vi "FP Server Repository.vi"(0 "FP Management In":refnum<class "Front Panel Manager.lvclass">, 5 "Action(ReadRepository)":T1(ring), 11 "error in (no error)":errorcluster) -> (4 "FP Management Out":refnum<class "Front Panel Manager.lvclass">, 6 "ToProcessQueue":refnum<queue>, 8 "ProcessAlreadyStarted":bool, 12 "ProcessViRef":refnum<vi>, 13 "ProcessSyncQueue":refnum<queue>, 14 "FromProcessQueue":refnum<queue>, 15 "error out":errorcluster)   [LabVIEW 2017, in "Front Panel Publisher.lvlib" / "Front Panel Manager.lvclass"]
uses:
  Front Panel Manager.lvclass
  FP Server Message.ctl
  FP Server.ctl
  Front Panel Manager.lvclass/Front Panel Manager.ctl
panel:
  # "Use this indicator for sending messages to the Process VI"
  # "These indicators are used by the process VIs"
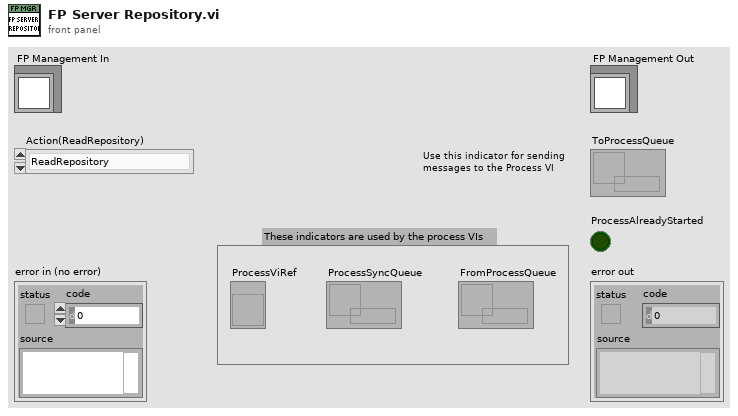
[diagram p1: front panel]
types:
  T1 = enum16{"ReadRepository", "CreateNew", "CreateOrLookUpExisting", "ReadRepositoryAndDestroy"}
  T2 = typedef "Front Panel Publisher.lvlib/Front Panel Manager.lvclass/FP Server.ctl" = cluster{"ToProcessQueue":refnum<queue>, "FromProcessQueue":refnum<queue>, "ProcessSyncQueue":refnum<queue>, "ProcessViRef":refnum<vi>}
  T3 = typedef "Front Panel Publisher.lvlib/Front Panel Manager.lvclass/FP Server Message.ctl" = cluster{"Message":string, "Page":string, "Data":string[][], "Connection ID":u64, "Values and Position":refnum<vi>[]}
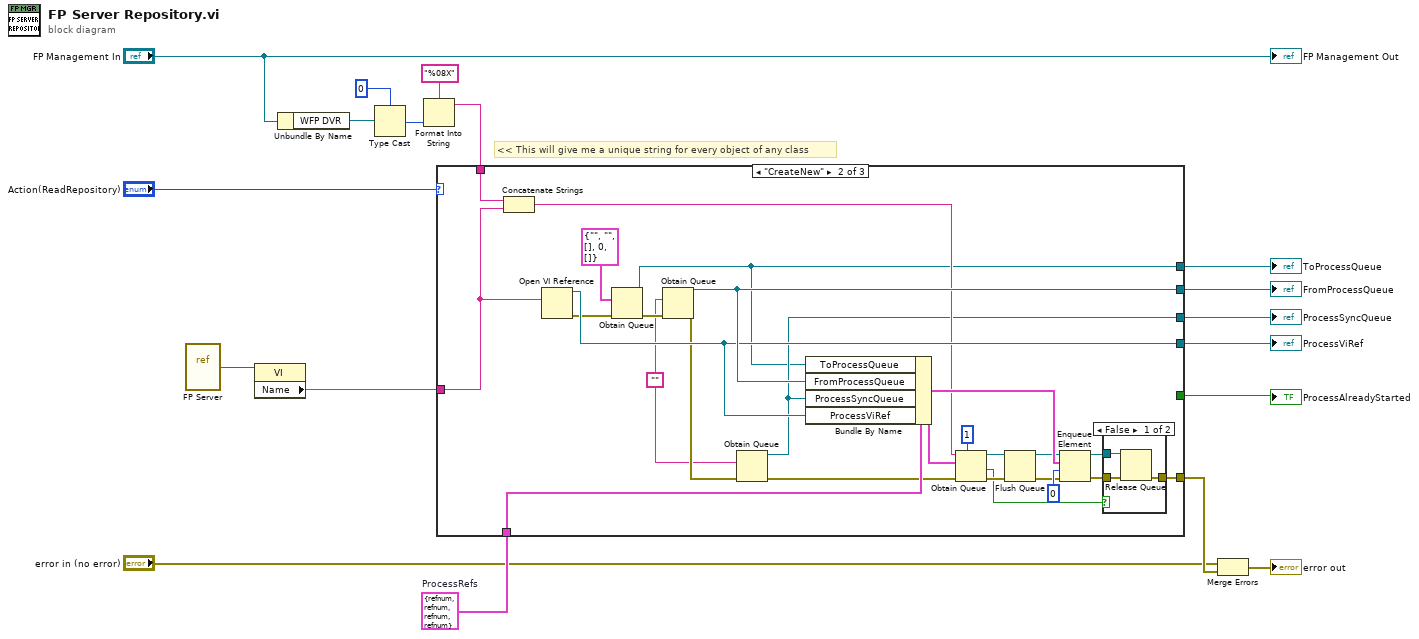
[diagram p0: block diagram]
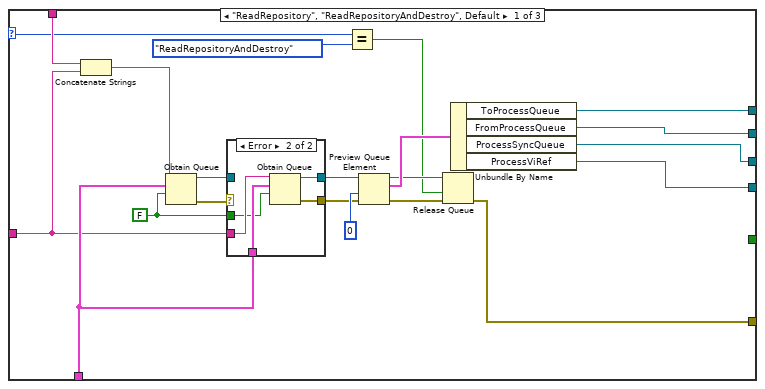
[diagram p2: hidden frame]
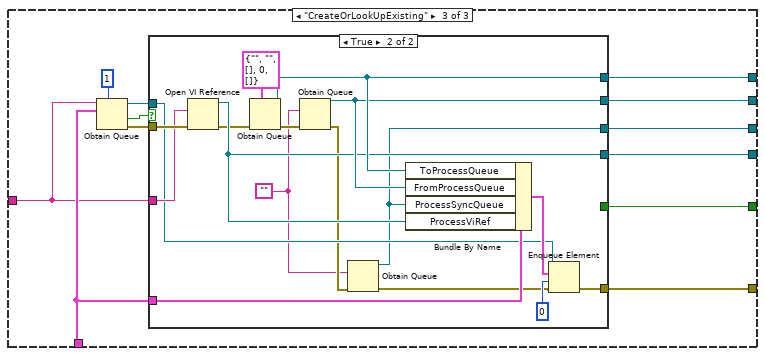
[diagram p5: hidden frame]
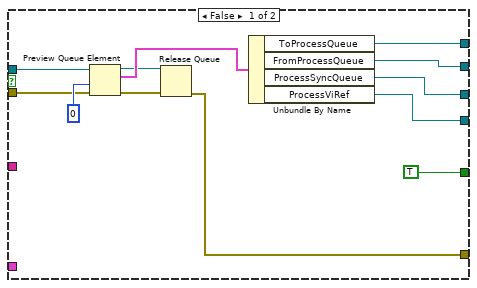
[diagram p6: hidden frame]
diagram:
  w13 = T2 {"ToProcessQueue"=refnum, "FromProcessQueue"=refnum, "ProcessSyncQueue"=refnum, "ProcessViRef"=refnum}  # ProcessRefs
  # "<< This will give me a unique string for every object of any class"
  n1 = vi-ref "FP Server.vi"() -> (w1:refnum<vi>)
  n2 = property class="VI"(reference=w1) -> ("Name"=w2:string)  [unwired: 1 in, 2 out]
  n3 = Unbundle By Name("FP Management In") -> ("WFP DVR"=w3:refnum<data-value>)
  n4 = Type Cast(type=u32 0, x=w3) -> (*(type *) &x=w8:u32)
  n5 = Format Into String(format string="%08X", w8) -> (resulting string=w5:string)  [unwired: 2 in, 1 out]
  n6 = case shown="\"CreateNew\"" "Action(ReadRepository)" {
    selector: "Action(ReadRepository)" -> [w20 _ _]
    tunnel: [w34 w57 w85] -> w17
    tunnel: [w36 w47 w87] -> w15
    tunnel: [w35 w71 w86] -> w16
    tunnel: [w37 w70 w84] -> w14
    tunnel: w13 -> [w29 w63 w80]
    tunnel: w5 -> [w27 w62 _]
    tunnel: [w22 w50 w83] -> w11
    tunnel: w2 -> [w26 w60 w76]
    tunnel: [_ _ w78] -> w10
    frame "ReadRepository", "ReadRepositoryAndDestroy", Default {
      w28 = FALSE ("create if not found? (T)")
      n7 = Concatenate Strings(w27, w26) -> (w25:string)
      n8 = Obtain Queue(name (unnamed)=w25, element data type=w29, create if not found? (T)=w28) -> (queue out=w31:refnum<queue>, error out=w33:errorcluster)  [unwired: 2 in, 1 out]
      n9 = case shown="Error" w33 {
        selector: w33 -> [w41 _]
        tunnel: [w41 w43] -> w32
        tunnel: w31 -> [w40 _]
        tunnel: [w40 w44] -> w30
        tunnel: w29 -> [_ w46]
        tunnel: w26 -> [_ w45]
        tunnel: w28 -> [_ w42]
        frame No Error {
        }
        frame Error {
          n10 = Obtain Queue(name (unnamed)=w45, element data type=w46, create if not found? (T)=w42) -> (queue out=w44:refnum<queue>, error out=w43:errorcluster)  [unwired: 2 in, 1 out]
        }
      }
      n11 = Equal?(x=w20, y=T1."ReadRepositoryAndDestroy") -> (x = y?=w19:bool)
      n12 = Preview Queue Element(queue=w30, timeout in ms (-1)=0, error in (no error)=w32) -> (queue out=w24:refnum<queue>, element=w38:T2, error out=w23:errorcluster)  [unwired: 1 out]
      n13 = Release Queue(queue=w24, force destroy? (F)=w19, error in (no error)=w23) -> (error out=w22:errorcluster)  [unwired: 2 out]
      n14 = Unbundle By Name(w38) -> ("ToProcessQueue"=w36:refnum<queue>, "FromProcessQueue"=w35:refnum<queue>, "ProcessSyncQueue"=w34:refnum<queue>, "ProcessViRef"=w37:refnum<vi>)
    }
    frame "CreateNew" {
      w56 = ""
      n15 = Concatenate Strings(w62, w60) -> (w61:string)
      n16 = Open VI Reference(vi path=w60) -> (vi reference=w70:refnum<vi>, error out=w68:errorcluster)  [unwired: 5 in]
      n17 = Obtain Queue(element data type=T3 {"Message"="", "Page"="", "Data"=[], "Connection ID"=0, "Values and Position"=[]} ("Process Message"), error in (no error)=w68) -> (queue out=w47:refnum<queue>, error out=w69:errorcluster)  [unwired: 3 in, 1 out]
      n18 = Obtain Queue(element data type=w56, error in (no error)=w69) -> (queue out=w71:refnum<queue>, error out=w59:errorcluster)  [unwired: 3 in, 1 out]
      n19 = Obtain Queue(element data type=w56, error in (no error)=w59) -> (queue out=w57:refnum<queue>, error out=w58:errorcluster)  [unwired: 3 in, 1 out]
      n20 = Bundle By Name(cluster=w63, "ToProcessQueue"=w47, "FromProcessQueue"=w71, "ProcessSyncQueue"=w57, "ProcessViRef"=w70) -> (w66:T2)
      n21 = Obtain Queue(max queue size (-1, unlimited)=1, name (unnamed)=w61, element data type=w66, error in (no error)=w58) -> (queue out=w67:refnum<queue>, created new?=w49:bool, error out=w54:errorcluster)  [unwired: 1 in]
      n22 = Flush Queue(queue=w67, error in (no error)=w54) -> (queue out=w55:refnum<queue>, error out=w53:errorcluster)  [unwired: 1 out]
      n23 = Enqueue Element(queue=w55, element=w66, timeout in ms (-1)=0, error in (no error)=w53) -> (queue out=w52:refnum<queue>, error out=w51:errorcluster)  [unwired: 1 out]
      n24 = case shown="False" w49 {
        tunnel: w51 -> [w74 w75]
        tunnel: w52 -> [w73 _]
        tunnel: [w72 w75] -> w50
        frame False {
          n25 = Release Queue(queue=w73, error in (no error)=w74) -> (error out=w72:errorcluster)  [unwired: 1 in, 2 out]
        }
        frame True {
        }
      }
    }
    frame "CreateOrLookUpExisting" {
      n26 = Obtain Queue(max queue size (-1, unlimited)=1, name (unnamed)=w76, element data type=w80) -> (queue out=w81:refnum<queue>, created new?=w82:bool, error out=w79:errorcluster)  [unwired: 2 in]
      n27 = case shown="True" w82 {
        tunnel: [w99 w116] -> w87
        tunnel: [w98 w115] -> w86
        tunnel: [w97 w101] -> w85
        tunnel: [w96 w114] -> w84
        tunnel: [w88 w113] -> w83
        tunnel: w80 -> [_ w112]
        tunnel: w79 -> [w93 w107]
        tunnel: w76 -> [_ w106]
        tunnel: w81 -> [w94 w105]
        tunnel: [TRUE _] -> w78
        frame False {
          n28 = Preview Queue Element(queue=w94, timeout in ms (-1)=0, error in (no error)=w93) -> (queue out=w90:refnum<queue>, element=w92:T2, error out=w89:errorcluster)  [unwired: 1 out]
          n29 = Release Queue(queue=w90, error in (no error)=w89) -> (error out=w88:errorcluster)  [unwired: 1 in, 2 out]
          n30 = Unbundle By Name(w92) -> ("ToProcessQueue"=w99:refnum<queue>, "FromProcessQueue"=w98:refnum<queue>, "ProcessSyncQueue"=w97:refnum<queue>, "ProcessViRef"=w96:refnum<vi>)
        }
        frame True {
          w102 = ""
          n31 = Open VI Reference(vi path=w106, error in (no error)=w107) -> (vi reference=w114:refnum<vi>, error out=w110:errorcluster)  [unwired: 4 in]
          n32 = Obtain Queue(element data type=T3 {"Message"="", "Page"="", "Data"=[], "Connection ID"=0, "Values and Position"=[]} ("Process Message"), error in (no error)=w110) -> (queue out=w116:refnum<queue>, error out=w111:errorcluster)  [unwired: 3 in, 1 out]
          n33 = Obtain Queue(element data type=w102, error in (no error)=w111) -> (queue out=w115:refnum<queue>, error out=w104:errorcluster)  [unwired: 3 in, 1 out]
          n34 = Obtain Queue(element data type=w102, error in (no error)=w104) -> (queue out=w101:refnum<queue>, error out=w103:errorcluster)  [unwired: 3 in, 1 out]
          n35 = Bundle By Name(cluster=w112, "ToProcessQueue"=w116, "FromProcessQueue"=w115, "ProcessSyncQueue"=w101, "ProcessViRef"=w114) -> (w109:T2)
          n36 = Enqueue Element(queue=w105, element=w109, timeout in ms (-1)=0, error in (no error)=w103) -> (error out=w113:errorcluster)  [unwired: 2 out]
        }
      }
    }
  }
  "ProcessSyncQueue" <- w17
  "ToProcessQueue" <- w15
  "FromProcessQueue" <- w16
  "ProcessViRef" <- w14
  "ProcessAlreadyStarted" <- w10
  n37 = Merge Errors("error in (no error)", w11) -> (→"error out":errorcluster)
  "FP Management Out" <- "FP Management In"
